vi "Start Command.vi"(8 "error in (no error)":errorcluster, 11 "Command in":refnum<class "Grab.lvclass">) -> (0 "error out":errorcluster, 3 "Command out":refnum<class "Grab.lvclass">)   [LabVIEW 2014, in "Grabber.lvlib" / "Grab.lvlib" / "Grab.lvclass"]
uses:
  Grab.lvclass
  Robot Actor Framework/Command Actor/Command Actor Messages/FInished Command Msg/Finish Command Msg.lvclass
  <vilib>/ActorFramework/Actor/Actor.lvclass/Actor.ctl
  <vilib>/ActorFramework/Message Enqueuer/Message Enqueuer.lvclass/Message Enqueuer.ctl
  <vilib>/ActorFramework/Message Enqueuer/Init from Existing Queue.vi
  <vilib>/ActorFramework/Message Enqueuer/Enqueue.vi
  <vilib>/ActorFramework/Message Priority Queue/Priority Enqueue.vi
  <vilib>/ActorFramework/Message Enqueuer/Message Enqueuer.lvclass
  Grabber Messages/Close Arms Msg/Close Arms Msg.lvclass
  Robot Actor Framework/Command Actor/Command Actor Class/Command Actor.lvclass
  <vilib>/ActorFramework/Actor/Actor.lvclass
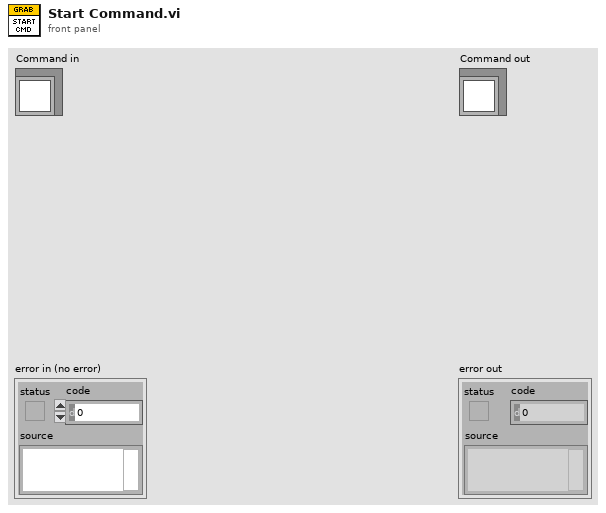
[diagram p1: front panel]
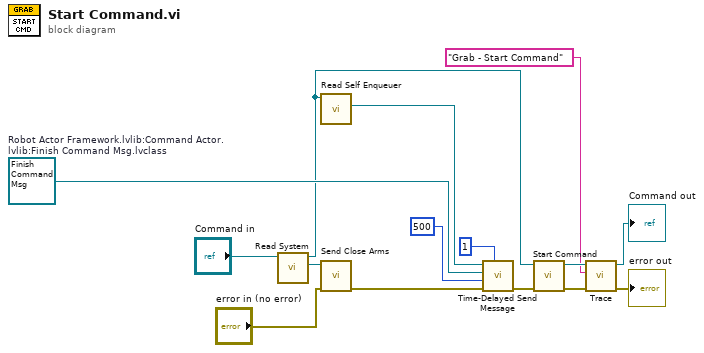
[diagram p0: block diagram]
diagram:
  w11 = refnum<class "Finish Command Msg.lvclass"> refnum  # Robot Actor Framework.lvlib:Command Actor.lvlib:Finish Command Msg.lvclass
  n1 = call-dynamic "Read System.vi"("Command in"="Command in") -> ("Actor Framework:Message Enqueuer"=w1:refnum<class "Message Enqueuer.lvclass">, "Command out"=w2:refnum<class "Grab.lvclass">)  [unwired: 8 in, 1 out]
  n2 = call <vilib>:"Read Self Enqueuer.vi"("Actor"=w2) -> ("Self Enqueuer"=w12:refnum<class "Message Enqueuer.lvclass">)  [unwired: 10 in]
  n3 = call "Send Close Arms.vi"("error in (no error)"="error in (no error)", "Message Enqueuer"=w1) -> ("error out"=w15:errorcluster)  [unwired: 8 in, 1 out]
  n4 = call <vilib>:"Time-Delayed Send Message.vi"("# Copies (0 = infinite repeat)"=u32 1, "error in (no error)"=w15, "Milliseconds To Wait"=500, "Message"=w11, "Message Enqueuer"=w12) -> ("error out"=w13:errorcluster)  [unwired: 5 in, 1 out]
  n5 = call-parent "Start Command.vi"("error in (no error)"=w13, "Command in"=w2) -> ("error out"=w6:errorcluster, "Command out"=w8:refnum<class "Grab.lvclass">)  [unwired: 8 in]
  n6 = call-dynamic "Trace.vi"("error in (no error)"=w6, "Command Action"="Grab - Start Command", "Command Actor in"=w8) -> ("error out"=→"error out":errorcluster, "Command Actor out"=→"Command out":refnum<class "Grab.lvclass">)  [unwired: 7 in]
